vi "Extract.vi"(8 "error in (no error)":errorcluster, 10 "AbstractData in":refnum<class "AbstractData.lvclass">, 11 "AbstractExtractor1D in":refnum<class "AbstractExtractor1D.lvclass">) -> (0 "error out":errorcluster, 3 "AbstractExtractor1D out":refnum<class "AbstractExtractor1D.lvclass">)   [LabVIEW 2014, in "AbstractExtractor1D.lvclass"]
uses:
  AbstractExtractor1D.lvclass
  Model/Data/AbstractData/AbstractData.lvclass
  Model/Data/Data1D/Data1D.lvclass
  AbstractExtractor/AbstractExtractor.lvclass
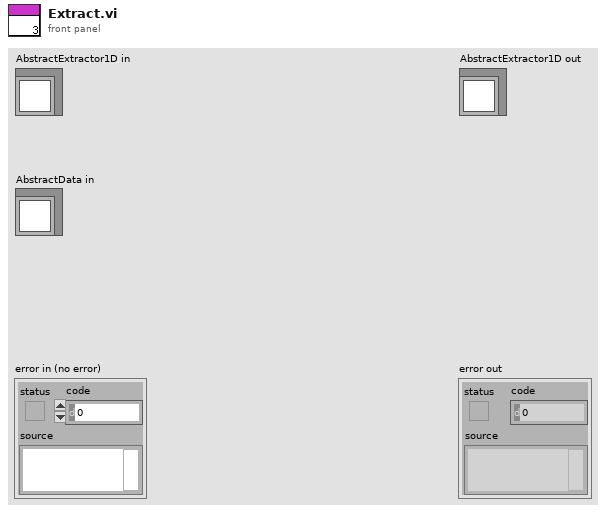
[diagram p1: front panel]
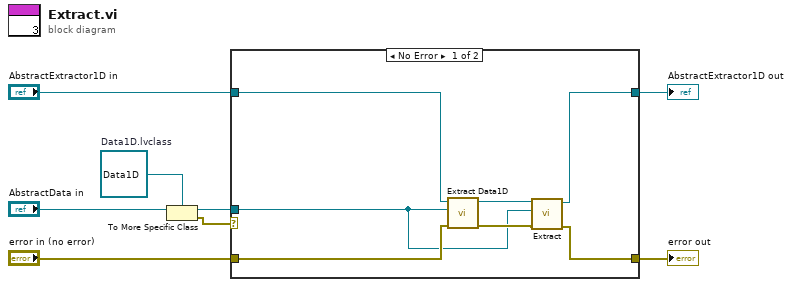
[diagram p0: block diagram]
diagram:
  w7 = refnum<class "Data1D.lvclass"> refnum  # Data1D.lvclass
  n1 = To More Specific Class(target class=w7, reference="AbstractData in") -> (specific class reference=w5:refnum<class "Data1D.lvclass">, error out=w6:errorcluster)  [unwired: 1 in]
  n2 = case shown="No Error" w6 {
    tunnel: w5 -> [w9 _]
    tunnel: "error in (no error)" -> [w14 w17]
    tunnel: [w11 w17] -> w3
    tunnel: "AbstractExtractor1D in" -> [w15 w16]
    tunnel: [w10 w16] -> w1
    frame No Error {
      n3 = call-dynamic "Extract Data1D.vi"("error in (no error)"=w14, "Data1D in"=w9, "AbstractExtractor1D in"=w15) -> ("error out"=w12:errorcluster, "AbstractExtractor1D out"=w13:refnum<class "AbstractExtractor1D.lvclass">)  [unwired: 7 in]
      n4 = call-parent "Extract.vi"("error in (no error)"=w12, "AbstractData in"=w9, "AbstractExtractor in"=w13) -> ("error out"=w11:errorcluster, "AbstractExtractor out"=w10:refnum<class "AbstractExtractor1D.lvclass">)  [unwired: 7 in]
    }
    frame Error {
    }
  }
  "error out" <- w3
  "AbstractExtractor1D out" <- w1
